vi "SPARK Configure Follower Mode.vi"   [LabVIEW 2023]
doc: "Configure follower mode on the SPARK."
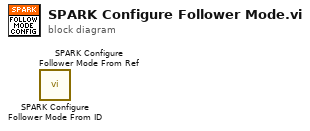
[diagram p0: block diagram]
diagram:
  n1 = call "SPARK Configure Follower Mode From ID.vi"() -> ()  [unwired: 10 in, 2 out]
  n2 = call "SPARK Configure Follower Mode From Ref.vi"() -> ()  [unwired: 10 in, 2 out]
